vi "aula1_eriton.vi"() -> ()   [LabVIEW 2024]
panel:
  in  "N":i32
  out "i":i32
  out "Meter":dbl(knob) scale=0.0..50.0
  out "element":dbl
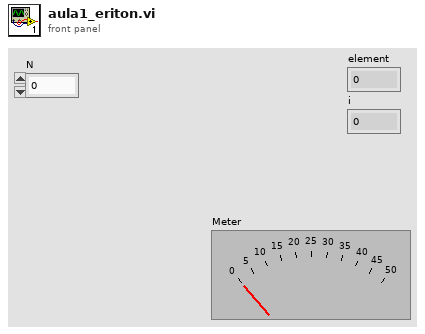
[diagram p1: front panel]
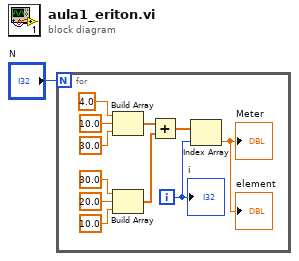
[diagram p0: block diagram]
diagram:
  n1 = for {
    N: "N" -> [_]
    i -> [w3]
    n2 = Build Array(4.0 ("element"), 10.0 ("element"), 30.0 ("element")) -> (w5:dbl[])
    n3 = Build Array(30.0 ("element"), 20.0 ("element"), 10.0 ("element")) -> (w6:dbl[])
    n4 = Add(x=w5, y=w6) -> (x+y=w4:dbl[])
    n5 = Index Array(array=w4, index=w3) -> (element=→"element" →"Meter":dbl)
    "i" <- w3
  }
